vi "1e6 div x(SubVI).vi"(11 "x":dbl) -> (3 "1e6/x":dbl)   [LabVIEW 2024]
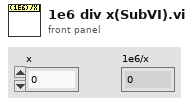
[diagram p1: front panel]
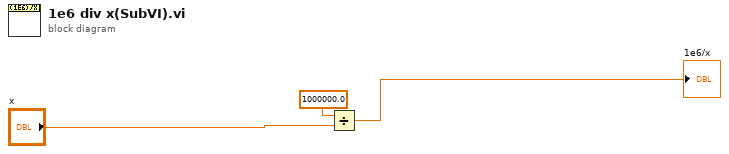
[diagram p0: block diagram]
diagram:
  n1 = Divide(x=1000000.0, y="x") -> (x/y=→"1e6/x":dbl)
